vi "读取配置.vi"() -> (0 "端口号":i32=8848, 1 "等待":i32=3000, 2 "当前城市":string="荆州", 3 "手动清扫周期":dbl=2.0, 4 "手动清扫速度":i32=1, 5 "清扫模式选择开关":bool, 6 "晴类清扫周期":dbl=2.0, 7 "阴类清扫周期":dbl=2.0, 8 "雨类清扫周期":dbl=2.0, 9 "雪类清扫周期":dbl=2.0, 10 "沙尘类清扫周期":dbl=2.0, 11 "其他类清扫周期":dbl=2.0, 12 "晴类清扫速度":i32=1, 13 "阴类清扫速度":i32=1, 14 "雨类清扫速度":i32=1, 15 "雪类清扫速度":i32=1, 16 "沙尘类清扫速度":i32=1, 17 "其他类清扫速度":i32=1)   [LabVIEW 2016]
uses:
  <vilib>/Utility/config.llb/Read Key (I32).vi
  <vilib>/Utility/config.llb/Read Key (String).vi
  <vilib>/Utility/config.llb/Read Key (Double).vi
  <vilib>/Utility/config.llb/Read Key (Boolean).vi
  <vilib>/Utility/config.llb/NI_LVConfig.lvlib
panel:
  out "error out":errorcluster caption="错误输出"
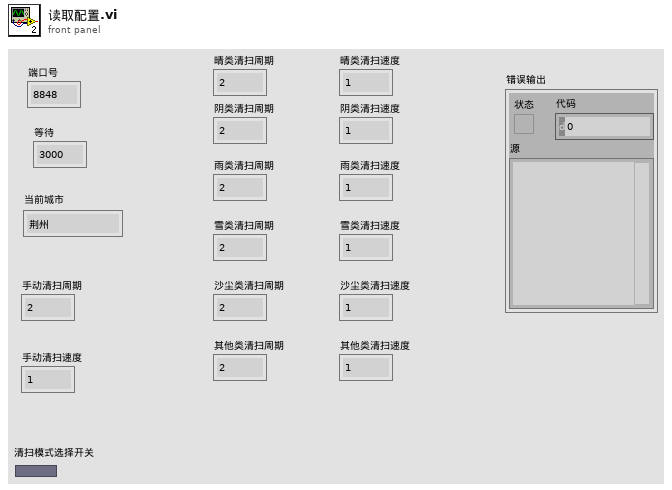
[diagram p1: front panel]
types:
  T1 = typedef "NI_LVConfig.lvlib/Config Data RefNum.ctl" = refnum<k1>
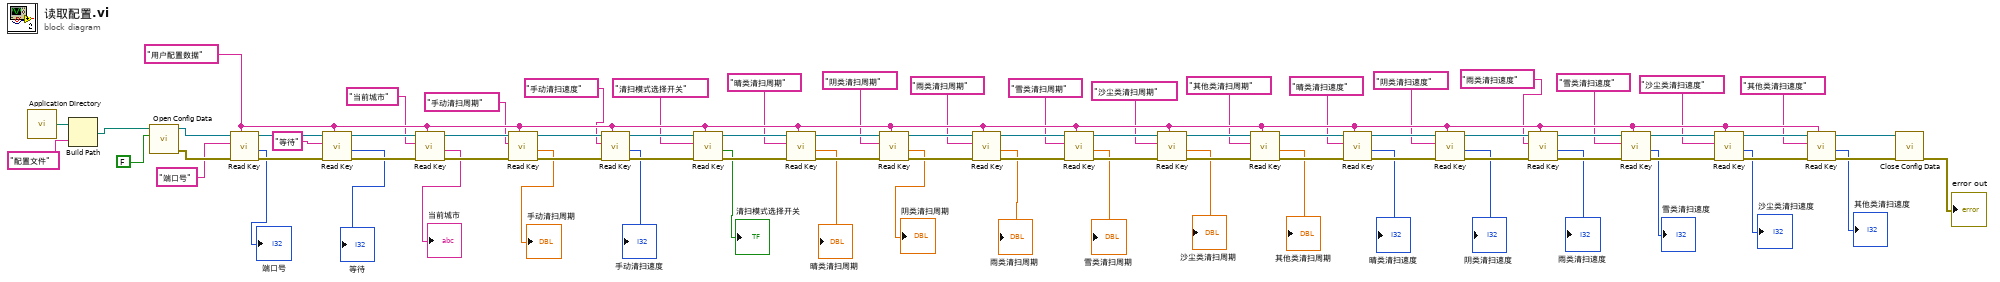
[diagram p0: block diagram]
diagram:
  w38 = "用户配置数据" ("section")
  n1 = call <vilib>:"Application Directory.vi"() -> ("Application Directory"=w79:path)
  n2 = Build Path(base path=w79, name or relative path="配置文件" ("名称或相对路径")) -> (appended path=w77:path)
  n3 = call <vilib>:"Open Config Data.vi"("create file if necessary (T)"=FALSE, "configuration file path"=w77) -> ("error out"=w37:errorcluster, "refnum"=w75:T1)  [unwired: 7 in, 1 out]
  n4 = call-poly <vilib>:"Read Key.vi"("section"=w38, "error in (no error)"=w37, "key"="端口号", "refnum"=w75) -> ("error out"=w70:errorcluster, "value"=→"端口号":i32, "refnum out"=w74:T1)  [unwired: 4 in, 1 out]
  n5 = call-poly <vilib>:"Read Key.vi"("section"=w38, "error in (no error)"=w70, "key"="等待", "refnum"=w74) -> ("error out"=w69:errorcluster, "value"=→"等待":i32, "refnum out"=w73:T1)  [unwired: 4 in, 1 out]
  n6 = call-poly <vilib>:"Read Key.vi"("section"=w38, "error in (no error)"=w69, "key"="当前城市", "refnum"=w73) -> ("error out"=w68:errorcluster, "value"=→"当前城市":string, "refnum out"=w72:T1)  [unwired: 4 in, 1 out]
  n7 = call-poly <vilib>:"Read Key.vi"("section"=w38, "error in (no error)"=w68, "key"="手动清扫周期", "refnum"=w72) -> ("error out"=w67:errorcluster, "value"=→"手动清扫周期":dbl, "refnum out"=w71:T1)  [unwired: 4 in, 1 out]
  n8 = call-poly <vilib>:"Read Key.vi"("section"=w38, "error in (no error)"=w67, "key"="手动清扫速度", "refnum"=w71) -> ("error out"=w66:errorcluster, "value"=→"手动清扫速度":i32, "refnum out"=w65:T1)  [unwired: 4 in, 1 out]
  n9 = call-poly <vilib>:"Read Key.vi"("section"=w38, "error in (no error)"=w66, "key"="清扫模式选择开关", "refnum"=w65) -> ("error out"=w63:errorcluster, "value"=→"清扫模式选择开关":bool, "refnum out"=w64:T1)  [unwired: 4 in, 1 out]
  n10 = call-poly <vilib>:"Read Key.vi"("section"=w38, "error in (no error)"=w63, "key"="晴类清扫周期", "refnum"=w64) -> ("error out"=w61:errorcluster, "value"=→"晴类清扫周期":dbl, "refnum out"=w62:T1)  [unwired: 4 in, 1 out]
  n11 = call-poly <vilib>:"Read Key.vi"("section"=w38, "error in (no error)"=w61, "key"="阴类清扫周期", "refnum"=w62) -> ("error out"=w59:errorcluster, "value"=→"阴类清扫周期":dbl, "refnum out"=w60:T1)  [unwired: 4 in, 1 out]
  n12 = call-poly <vilib>:"Read Key.vi"("section"=w38, "error in (no error)"=w59, "key"="雨类清扫周期", "refnum"=w60) -> ("error out"=w57:errorcluster, "value"=→"雨类清扫周期":dbl, "refnum out"=w58:T1)  [unwired: 4 in, 1 out]
  n13 = call-poly <vilib>:"Read Key.vi"("section"=w38, "error in (no error)"=w57, "key"="雪类清扫周期", "refnum"=w58) -> ("error out"=w55:errorcluster, "value"=→"雪类清扫周期":dbl, "refnum out"=w56:T1)  [unwired: 4 in, 1 out]
  n14 = call-poly <vilib>:"Read Key.vi"("section"=w38, "error in (no error)"=w55, "key"="沙尘类清扫周期", "refnum"=w56) -> ("error out"=w53:errorcluster, "value"=→"沙尘类清扫周期":dbl, "refnum out"=w54:T1)  [unwired: 4 in, 1 out]
  n15 = call-poly <vilib>:"Read Key.vi"("section"=w38, "error in (no error)"=w53, "key"="其他类清扫周期", "refnum"=w54) -> ("error out"=w51:errorcluster, "value"=→"其他类清扫周期":dbl, "refnum out"=w52:T1)  [unwired: 4 in, 1 out]
  n16 = call-poly <vilib>:"Read Key.vi"("section"=w38, "error in (no error)"=w51, "key"="晴类清扫速度", "refnum"=w52) -> ("error out"=w49:errorcluster, "value"=→"晴类清扫速度":i32, "refnum out"=w50:T1)  [unwired: 4 in, 1 out]
  n17 = call-poly <vilib>:"Read Key.vi"("section"=w38, "error in (no error)"=w49, "key"="阴类清扫速度", "refnum"=w50) -> ("error out"=w47:errorcluster, "value"=→"阴类清扫速度":i32, "refnum out"=w48:T1)  [unwired: 4 in, 1 out]
  n18 = call-poly <vilib>:"Read Key.vi"("section"=w38, "error in (no error)"=w47, "key"="雨类清扫速度", "refnum"=w48) -> ("error out"=w45:errorcluster, "value"=→"雨类清扫速度":i32, "refnum out"=w46:T1)  [unwired: 4 in, 1 out]
  n19 = call-poly <vilib>:"Read Key.vi"("section"=w38, "error in (no error)"=w45, "key"="雪类清扫速度", "refnum"=w46) -> ("error out"=w43:errorcluster, "value"=→"雪类清扫速度":i32, "refnum out"=w44:T1)  [unwired: 4 in, 1 out]
  n20 = call-poly <vilib>:"Read Key.vi"("section"=w38, "error in (no error)"=w43, "key"="沙尘类清扫速度", "refnum"=w44) -> ("error out"=w41:errorcluster, "value"=→"沙尘类清扫速度":i32, "refnum out"=w42:T1)  [unwired: 4 in, 1 out]
  n21 = call-poly <vilib>:"Read Key.vi"("section"=w38, "error in (no error)"=w41, "key"="其他类清扫速度", "refnum"=w42) -> ("error out"=w39:errorcluster, "value"=→"其他类清扫速度":i32, "refnum out"=w40:T1)  [unwired: 4 in, 1 out]
  n22 = call <vilib>:"Close Config Data.vi"("error in (no error)"=w39, "refnum"=w40) -> ("error out"=→"error out":errorcluster)  [unwired: 8 in, 1 out]
